vi "SaveEYE_RT_Single.vi"(4 "Motion Settings":T1={"No Motion?"=FALSE, "Motion System"=enum."NI 735x", "Motion Bd ID"=1, "Motion Profile"="SMAC1", "# Axis"=1, "Reverse Z axis?"=TRUE, "SMAC Axis"=0, "scan pair"=enum."y-(x) scan", "RT fps"=6.0, "Steps per mm"=[1000, 1000, 1000, 1000], "Motor Parameters"={"velocity ct/s"=[10000.0, 10000.0, 10000.0, 50000.0], "accel ct/s^2"=[50000.0, 50000.0, 50000.0, 200000.0]}, "One Way Scan"=FALSE, "Reverse One Way Scan"=FALSE, "Global Position (mm)"=[], "Plane"=0, "Distance between\nscan lines (um)"=0.0, "Distance between\nscan planes (um)"=0.0, "number of scan planes"=1, "Total steps in line"=0, "Xtra plane\ndistance  (um)"=100, "Xtra planes "=1, "Add Axis"=FALSE, "overshoot cts"=200, "BKPT Shift"=0, "Scan Start Time (ms)"=0, "ESP VISA"="GPIB::1::INSTR", "3rd Axis"=1, "GL Ref Out"=refnum, "Galil Address"=""} {"3rd Axis" items=["x", "y", "z", "w"]; "Xtra planes" min=1; "Xtra plane\ndistance  (um)" min=0; "Distance between\nscan planes (um)" format="%.2f"; "Distance between\nscan lines (um)" format="%.2f"; "SMAC Axis" items=["None"=0, "Axis 1"=1, "Axis 2"=2, "Axis 3"=3, "Axis 4"=4, "Axis 5"=5, "Axis 6"=6, "Axis 7"=7, "Axis 8"=8, "Vector Space 1"=17, "Vector Space 2"=18, "Vector Space 3"=19, "Vector Space 4"=20]; "Motion Bd ID" min=1 max=32 step=1}, 5 "gain":dbl=1.0, 7 "*.eye":bool, 8 "Digitizer Settings":T5={"Digitizer delay (us) "=0.0, "rf points per line"=2048, "lines per plane"=128, "Samp Rate (Hz)"=100000000.0, "Additional dig delay (us)"=0.0, "Voltage Scale"=0.4, "Pre-Looks"=0, "Offset delay (us)"=0.0, "bits A/D"=8, "Avg Num"=1, "DigTimeOut"=5.0, "Rel Dig Delay"=0.0, "Dig Ch"=0, "LeCroyCluster"={"LeCroy Channels"=[TRUE, FALSE, FALSE, FALSE], "LC read pt offset"=0.0, "Sweep Avg"=FALSE}, "Main Digitizer"=enum."NI Digitizer", "Dig Config"=enum."Single channel", "Digitizer ID Cluster"={"Acqiris/Alazar/SP ID"=[], "NI Instr Handles"=[], "LeCroy VISA"="", "GaGe Handle"={"Handle"=0, "Sample size"=0, "Resolution"=0, "Offset"=0, "Channels"=0, "Boards"=0}, "ATS Ref"="ATS9350", "Acqiris Address"=["PCI::INSTR0"], "ADQRef"=refnum, "adq_cu_ptr"=refnum}, "Trigger Settings"={"Trig Source"=1, "Trig Coupling"=0, "Trig Slope"=0, "Level (mV)"=1500.0}, "Bulk Acq"=FALSE, "Bulk Start Indexes"=[], "Data Ref RF"=refnum, "NI ID/Channel"=[], "Total Dig CH"=1, "Xtra Ann Trig delay (us)"=10.0, "Fix Z Delay?"=FALSE, "One Way Transmission?"=FALSE, "Data Ref Log"=refnum} {"Trigger Settings"."Trig Slope" items=["Positive", "Negative"]; "Trigger Settings"."Level (mV)" format="%.2f"; "Trigger Settings"."Trig Coupling" items=["DC 1 MOhm", "AC 1 MOhm", "DC 50 Ohm", "AC 50 Ohm"]; "Trigger Settings"."Trig Source" items=["Chan 1", "External"]; "Rel Dig Delay" format="%.2f"; "DigTimeOut" format="%.2f"; "Avg Num" min=1; "Offset delay (us)" format="%.2f"; "Additional dig delay (us)" format="%.2f"; "Digitizer delay (us)" format="%.2f"}, 9 "gain 2 Ch":dbl=1.0, 10 "Frame":i32, 11 "Data":i16[][](array[numeric])) -> ()   [LabVIEW 2022 SP3]
uses:
  ScanningControl/Digitizers/-DigitizerRoutines/DigitizerSettings.ctl
  ScanningControl/Digitizers/-DigitizerRoutines/Digitizer.ctl
  ScanningControl/Digitizers/-DigitizerRoutines/DigConfig.ctl
  ScanningControl/Digitizers/-DigitizerRoutines/DigitizerID.ctl
  C:/Windows/System32/ADQAPI_dotNet_helper.dll
  ScanningControl/Motion Controllers/NI_controller/-NI_MotionRoutines/MotionParameters.ctl
  ScanningControl/Motion Controllers/NI_controller/-NI_MotionRoutines/MotionSys.ctl
  ScanningControl/Motion Controllers/-MotionRoutines/ScanAxis.ctl
  ScanningControl/Motion Controllers/-MotionRoutines/3rdAxis.ctl
  ScanningControl/Motion Controllers/-MotionRoutines/MotionGlobals.vi
panel:
  in  "Movie Name":string="none"
  # "1-D and 2-D B scan settings"
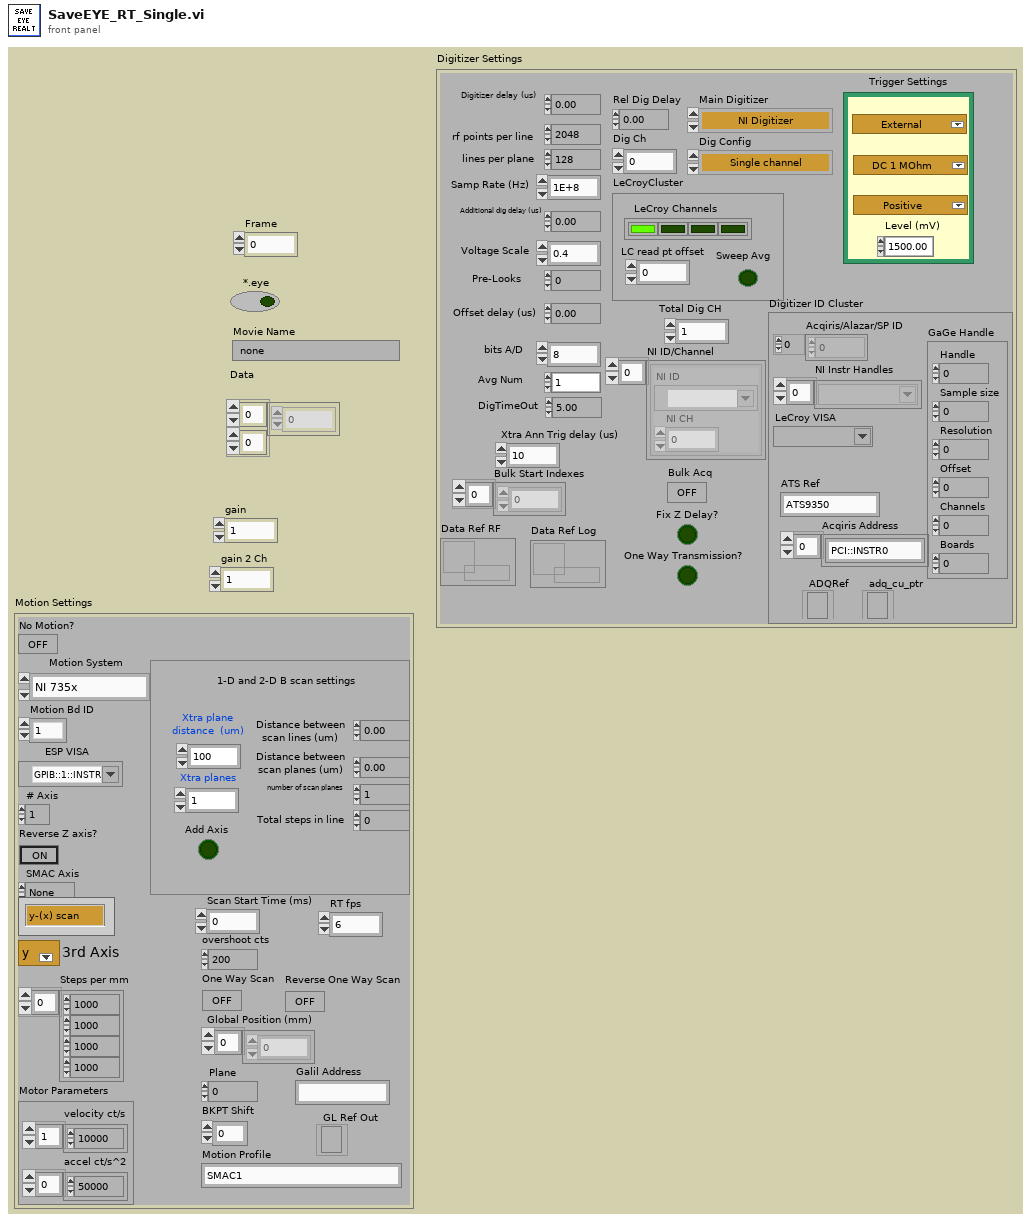
[diagram p1: front panel]
types:
  T1 = typedef "MotionParameters.ctl" = cluster{"No Motion?":bool, "Motion System":T2, "Motion Bd ID":u8, "Motion Profile":string, "# Axis":i8, "Reverse Z axis?":bool, "SMAC Axis":u16, "scan pair":T3, "RT fps":sgl, "Steps per mm":i32[], "Motor Parameters":cluster{"velocity ct/s":dbl[], "accel ct/s^2":dbl[]}, "One Way Scan":bool, "Reverse One Way Scan":bool, "Global Position (mm)":dbl[], "Plane":i32, "Distance between\nscan lines (um)":sgl, "Distance between\nscan planes (um)":sgl, "number of scan planes":i32, "Total steps in line":i32, "Xtra plane\ndistance  (um)":i32, "Xtra planes ":i32, "Add Axis":bool, "overshoot cts":i32, "BKPT Shift":i32, "Scan Start Time (ms)":u32, "ESP VISA":refnum<visa-resource-name>, "3rd Axis":T4, "GL Ref Out":refnum<k7>, "Galil Address":string}
  T2 = typedef "MotionSys.ctl" = enum16{"MM3000", "NI 735x", "Newport ESP", "No Motion Card", "Galil"}
  T3 = typedef "ScanAxis.ctl" = enum16{"y-(x) scan", "x-(y) scan", "z-(x) scan", "z-(y) scan", "y-(z) scan", "x-(z) scan", "w-(x) scan", "w-(y) scan", "w-(z) scan", "x-(w) scan", "y-(w) scan", "z-(w) scan"}
  T4 = typedef "3rdAxis.ctl" = u16
  T5 = typedef "DigitizerSettings.ctl" = cluster{"Digitizer delay (us) ":dbl, "rf points per line":i32, "lines per plane":i32, "Samp Rate (Hz)":dbl, "Additional dig delay (us)":dbl, "Voltage Scale":dbl, "Pre-Looks":i32, "Offset delay (us)":dbl, "bits A/D":i8, "Avg Num":i32, "DigTimeOut":sgl, "Rel Dig Delay":sgl, "Dig Ch":i32, "LeCroyCluster":cluster{"LeCroy Channels":bool[], "LC read pt offset":dbl, "Sweep Avg":bool}, "Main Digitizer":T6, "Dig Config":T7, "Digitizer ID Cluster":T8, "Trigger Settings":cluster{"Trig Source":u16, "Trig Coupling":u16, "Trig Slope":u16, "Level (mV)":dbl}, "Bulk Acq":bool, "Bulk Start Indexes":i32[], "Data Ref RF":refnum<data-value>, "NI ID/Channel":cluster{"NI ID":refnum<k15>, "NI CH":i32}[], "Total Dig CH":i32, "Xtra Ann Trig delay (us)":dbl, "Fix Z Delay?":bool, "One Way Transmission?":bool, "Data Ref Log":refnum<data-value>}
  T6 = typedef "Digitizer.ctl" = enum16{"Acqiris Digitizer", "NI Digitizer", "LeCroy", "GaGe", "AlazarTech", "No Digitizer", "Teledyne"}
  T7 = typedef "DigConfig.ctl" = enum16{"Single channel", "2 Chans w/ 2 Acqiris", "2 Chans w/ 1 Acqiris", "5-CH Pulser New", "5-CH pulser w/ ann array", "5-pass style ann array", "Empty"}
  T8 = typedef "DigitizerID.ctl" = cluster{"Acqiris/Alazar/SP ID":u32[], "NI Instr Handles":refnum<k15>[], "LeCroy VISA":refnum<visa-resource-name>, "GaGe Handle":cluster{"Handle":u32, "Sample size":u32, "Resolution":i32, "Offset":i32, "Channels":u32, "Boards":u32}, "ATS Ref":string, "Acqiris Address":string[], "ADQRef":refnum<k24>, "adq_cu_ptr":refnum<k24>}
  T9 = enum16{"open", "replace", "create", "open or create", "replace or create", "replace or create with confirmation"}
  T10 = enum16{"big-endian, network order", "native, host order", "little-endian"}
  T11 = cluster{"a":dbl, "Full Scale":dbl, "Full Scale":dbl}
  T12 = cluster{sgl, "Gain [dB]  ":sgl, "Atten (dB)":sgl}
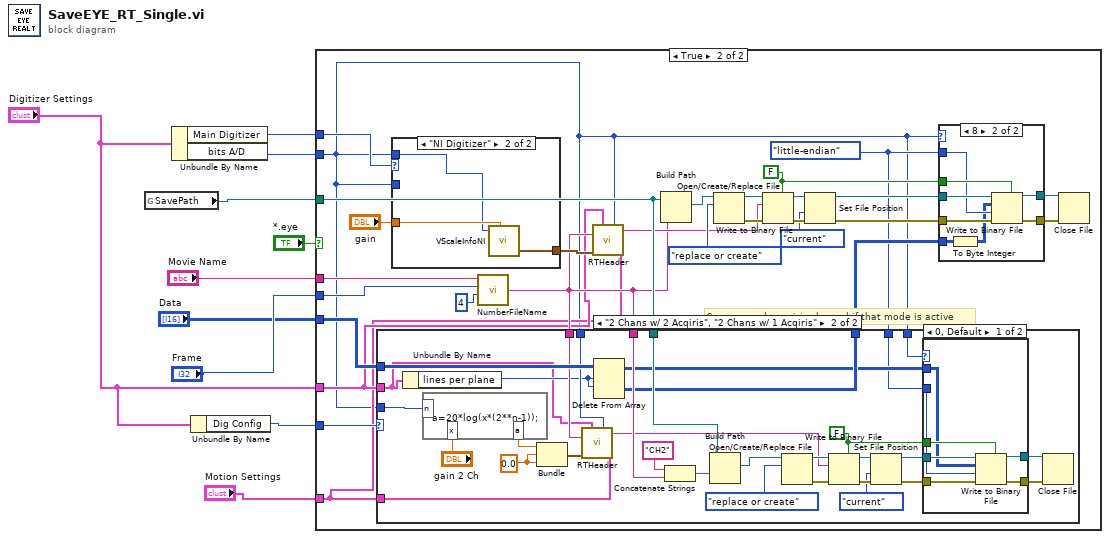
[diagram p0: block diagram]
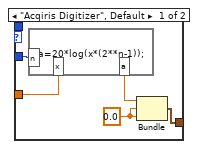
[diagram p3: hidden frame]
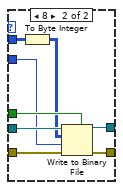
[diagram p5: hidden frame]
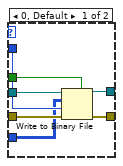
[diagram p6: hidden frame]
diagram:
  n1 = global read "MotionGlobals.vi" "SavePath"() -> (w7:path)
  n2 = Unbundle By Name("Digitizer Settings") -> ("Main Digitizer"=w4:T6, "bits A/D"=w5:i8)
  n3 = Unbundle By Name("Digitizer Settings") -> ("Dig Config"=w2:T7)
  n4 = case shown="True" "*.eye" {
    tunnel: "Data" -> [_ w20]
    tunnel: "Frame" -> [_ w38]
    tunnel: "Movie Name" -> [_ w37]
    tunnel: w7 -> [_ w19]
    tunnel: w2 -> [_ w22]
    tunnel: w5 -> [_ w11]
    tunnel: "Digitizer Settings" -> [_ w14]
    tunnel: w4 -> [_ w13]
    tunnel: "Motion Settings" -> [_ w12]
    frame False {
    }
    frame True {
      w15 = T10."little-endian" ("byte order (0:big-endian, network order)")
      w36 = FALSE ("prepend array or string size? (T)")
      # "Save second acquiris channel if that mode is active"
      n5 = case shown="\"NI Digitizer\"" w13 {
        tunnel: [w42 w46] -> w24
        tunnel: "gain" -> [w40 w45]
        tunnel: w11 -> [w39 _]
        tunnel: w11 -> [_ w44]
        frame "Acqiris Digitizer", Default {
          w43 = 0.0 ("Full Scale")
          n6 = formula code="a=20*log(x*(2**n-1));"("x"=w40, "n"=w39) -> ("a"=w41:dbl)
          n7 = Bundle("a"=w41, "Full Scale"=w43, "Full Scale"=w43) -> (w42:T11)  [unwired: 1 out]
        }
        frame "NI Digitizer" {
          n8 = call "VScaleInfoNI.vi"("A/D bits"=w44, "gain"=w45) -> ("Voltage Scale"=w46:T12)  [unwired: 5 in, 3 out]
        }
      }
      n9 = call "NumberFileName.vi"("Digits"=4, "File number"=w38, "file name"=w37) -> ("Numbered File"=w17:string)  [unwired: 1 in]
      n10 = case shown="\"2 Chans w/ 2 Acqiris\", \"2 Chans w/ 1 Acqiris\"" w22 {
        tunnel: [w47 w54] -> w21
        tunnel: w20 -> [w47 w62]
        tunnel: w17 -> [_ w67]
        tunnel: w19 -> [_ w64]
        tunnel: w11 -> [_ w63]
        tunnel: w17 -> [_ w59]
        tunnel: w11 -> [_ w58]
        tunnel: w15 -> [_ w52]
        tunnel: w11 -> [_ w51]
        tunnel: w14 -> [_ w49]
        tunnel: w12 -> [_ w48]
        frame "Single channel", Default {
        }
        frame "2 Chans w/ 2 Acqiris", "2 Chans w/ 1 Acqiris" {
          w61 = 0.0 ("Full Scale")
          w79 = FALSE ("prepend array or string size? (T)")
          n11 = Unbundle By Name(w49) -> ("lines per plane"=w50:i32)
          n12 = formula code="a=20*log(x*(2**n-1));"("x"="gain 2 Ch", "n"=w51) -> ("a"=w56:dbl)
          n13 = Bundle("a"=w56, "Full Scale"=w61, "Full Scale"=w61) -> (w60:T11)  [unwired: 1 out]
          n14 = call "RTHeader.vi"("Digitizer Settings"=w49, "Dig Word Size"=w58, "File Name In"=w59, "Votage scaling"=w60, "Motion Settings"=w48) -> ("Header String Out"=w57:string)  [unwired: 9 in, 1 out]
          n15 = Delete From Array(array=w62, length=w50, index (row)=w50) -> (deleted portion=w54:i16[][], array with subset deleted=w53:i16[][])  [unwired: 1 in]
          n16 = Concatenate Strings("CH2", w67) -> (w65:string)
          n17 = Build Path(base path=w64, name or relative path=w65) -> (appended path=w69:path)
          n18 = Open/Create/Replace File(file path (use dialog)=w69, operation (0:open)=T9."replace or create") -> (refnum out=w75:refnum<file>, error out=w76:errorcluster)  [unwired: 1 in, 4 out]
          n19 = Write to Binary File(file (use dialog)=w75, data=w57, error in=w76, 5:w79) -> (refnum out=w73:refnum<file>, error out=w74:errorcluster)  [unwired: 3 out]
          n20 = Set File Position(refnum=w73, from (0:start)=enum16{"start", "end", "current"}."current" ("pos mode (0:2)"), error in=w74) -> (refnum out=w77:refnum<file>, error out=w78:errorcluster)  [unwired: 1 out]
          n21 = case shown="0, Default" w63 {
            tunnel: w52 -> [w86 w89]
            tunnel: w79 -> [w85 w94]
            tunnel: w78 -> [w84 w93]
            tunnel: w77 -> [w83 w92]
            tunnel: [w82 w91] -> w71
            tunnel: [w81 w90] -> w70
            tunnel: w53 -> [w80 w87]
            frame 0, Default {
              n22 = Write to Binary File(file (use dialog)=w83, data=w80, error in=w84, 5:w85, 9:w86) -> (refnum out=w82:refnum<file>, error out=w81:errorcluster)  [unwired: 2 out]
            }
            frame 8 {
              n23 = To Byte Integer(number=w87) -> (8bit integer=w88:i8[][])
              n24 = Write to Binary File(file (use dialog)=w92, data=w88, error in=w93, 5:w94, 9:w89) -> (refnum out=w91:refnum<file>, error out=w90:errorcluster)  [unwired: 2 out]
            }
          }
          n25 = Close File(refnum=w71, error in=w70) -> ()  [unwired: 2 out]
        }
      }
      n26 = call "RTHeader.vi"("Digitizer Settings"=w14, "Dig Word Size"=w11, "File Name In"=w17, "Votage scaling"=w24, "Motion Settings"=w12) -> ("Header String Out"=w18:string)  [unwired: 9 in, 1 out]
      n27 = Build Path(base path=w19, name or relative path=w17) -> (appended path=w25:path)
      n28 = Open/Create/Replace File(file path (use dialog)=w25, operation (0:open)=T9."replace or create") -> (refnum out=w32:refnum<file>, error out=w33:errorcluster)  [unwired: 1 in, 4 out]
      n29 = Write to Binary File(file (use dialog)=w32, data=w18, error in=w33, 5:w36) -> (refnum out=w30:refnum<file>, error out=w31:errorcluster)  [unwired: 3 out]
      n30 = Set File Position(refnum=w30, from (0:start)=enum16{"start", "end", "current"}."current" ("pos mode (0:2)"), error in=w31) -> (refnum out=w34:refnum<file>, error out=w35:errorcluster)  [unwired: 1 out]
      n31 = case shown="8" w11 {
        tunnel: w15 -> [w101 w103]
        tunnel: w36 -> [w100 w109]
        tunnel: w35 -> [w99 w108]
        tunnel: w34 -> [w98 w107]
        tunnel: [w97 w106] -> w28
        tunnel: [w96 w105] -> w27
        tunnel: w21 -> [w95 w104]
        frame 0, Default {
          n32 = Write to Binary File(file (use dialog)=w98, data=w95, error in=w99, 5:w100, 9:w101) -> (refnum out=w97:refnum<file>, error out=w96:errorcluster)  [unwired: 2 out]
        }
        frame 8 {
          n33 = To Byte Integer(number=w104) -> (8bit integer=w102:i8[][])
          n34 = Write to Binary File(file (use dialog)=w107, data=w102, error in=w108, 5:w109, 9:w103) -> (refnum out=w106:refnum<file>, error out=w105:errorcluster)  [unwired: 2 out]
        }
      }
      n35 = Close File(refnum=w28, error in=w27) -> ()  [unwired: 2 out]
    }
  }
